vi "StatusUpdate.vi"(8 "error in (no error)":errorcluster, 9 "Status":string, 10 "ModuleID":i32) -> (0 "error out":errorcluster)   [LabVIEW 2018, in "FgenPlugins.lvlib"]
uses:
  FgenShared/clEventType.ctl
  FgenPlugins.lvlib
  FgenShared/FgenShared.lvlib
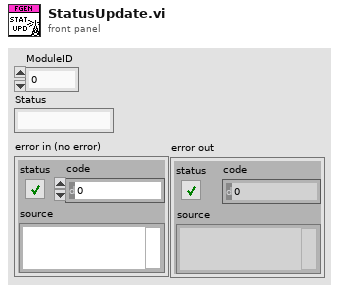
[diagram p1: front panel]
types:
  T1 = typedef "FgenShared.lvlib/clEventType.ctl" = cluster{"ModuleID":i32, "Data":variant}
  T2 = typedef "FgenShared.lvlib/clBroadcastEvents.ctl" = cluster{"DidInit":refnum<user-event>, "StatusUpdate":refnum<user-event>, "ErrorReport":refnum<user-event>, "DidStop":refnum<user-event>, "PathToINI":refnum<user-event>, "Channels":refnum<user-event>, "Function":refnum<user-event>, "Waveforms":refnum<user-event>, "Triggers":refnum<user-event>, "FunctionParams":refnum<user-event>, "FunctionArbs":refnum<user-event>, "FunctionSampleRate":refnum<user-event>}
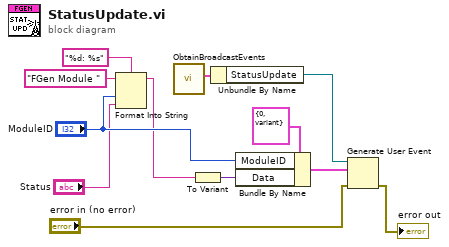
[diagram p0: block diagram]
diagram:
  n1 = Format Into String(format string="%d: %s", initial string="FGen Module ", "ModuleID", "Status") -> (resulting string=w1:string)  [unwired: 1 in, 1 out]
  n2 = call "ObtainBroadcastEvents.vi"() -> ("clBroadcastEvents"=w12:T2)  [unwired: 10 in, 1 out]
  n3 = To Variant(anything=w1) -> (Variant=w9:variant)
  n4 = Unbundle By Name(w12) -> ("StatusUpdate"=w11:refnum<user-event>)
  n5 = Bundle By Name(cluster=T1 {"ModuleID"=0, "Data"=variant} ("clBroadcast"), "ModuleID"="ModuleID", "Data"=w9) -> (w8:T1)
  n6 = Generate User Event(user event=w11, event data cluster=w8, error in="error in (no error)") -> (error out=→"error out":errorcluster)  [unwired: 1 in, 1 out]
